vi "Write Attributes.vi"(8 "error in (no error)":errorcluster, 10 "Attributes":refnum<class "Attribute.lvclass">[](array[class]), 11 "Reference in":refnum<class "Reference.lvclass">) -> (0 "error out":errorcluster, 3 "Reference out":refnum<class "Reference.lvclass">)   [LabVIEW 2018, in "VILab.lvlib" / "Reference.lvclass"]
uses:
  Reference.lvclass
  Attribute.lvclass
  <vilib>/Utility/error.llb/Error Cluster From Error Code.vi
  <vilib>/ErrorRing/Error Ring.xnode
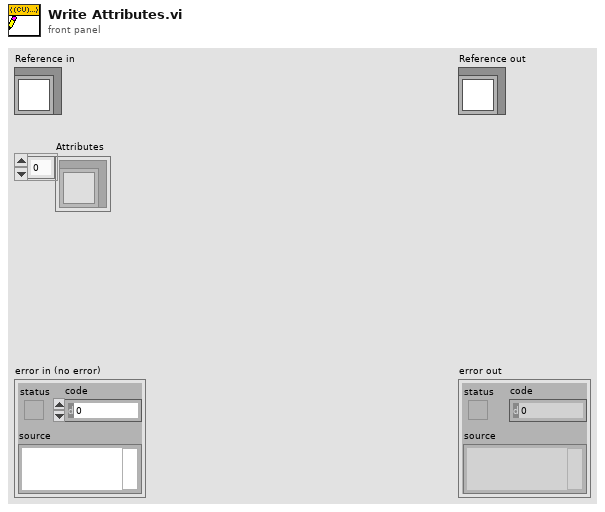
[diagram p1: front panel]
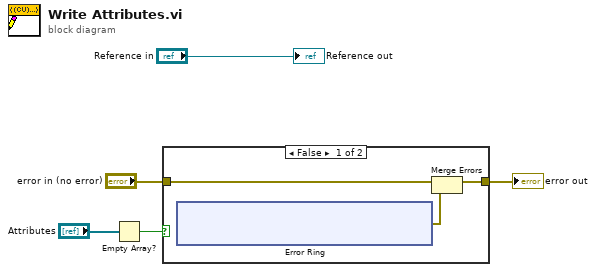
[diagram p0: block diagram]
diagram:
  n1 = Empty Array?(array="Attributes") -> (empty?=w1:bool)
  n2 = case shown="False" w1 {
    tunnel: "error in (no error)" -> [w8 w13]
    tunnel: [w7 w13] -> w3
    frame False {
      n3 = xnode "Error Ring"() -> ("error out"=w6:errorcluster)
      n4 = Merge Errors(w8, w6) -> (w7:errorcluster)
    }
    frame True {
    }
  }
  "error out" <- w3
  "Reference out" <- "Reference in"
